vi "Measurement.UI.SetControllerDependency.vi"(8 "error in (no error)":errorcluster, 10 "Measurement":refnum<class "Measurement.lvclass">, 11 "Measurement.PhotocurrentMapping.UI in":refnum<class "Measurement.PhotocurrentMapping.UI.lvclass">) -> (0 "error out":errorcluster, 3 "Measurement.PhotocurrentMapping.UI out":refnum<class "Measurement.PhotocurrentMapping.UI.lvclass">)   [LabVIEW 2019, in "Measurement.PhotocurrentMapping.UI.lvclass"]
uses:
  Measurement.PhotocurrentMapping.UI.lvclass
  Measurement/Measurement.lvclass
  Measurement.PhotocurrentMapping/Measurement.PhotocurrentMapping.lvclass
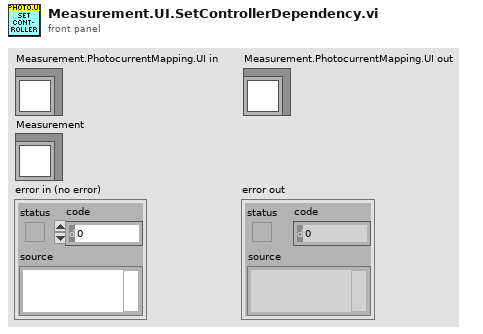
[diagram p1: front panel]
types:
  T1 = typedef "Measurement.PhotocurrentMapping.UI.lvclass/Dependencies--Cluster.ctl" = cluster{"Measurement.PhotocurrentMapping":refnum<class "Measurement.PhotocurrentMapping.lvclass">}
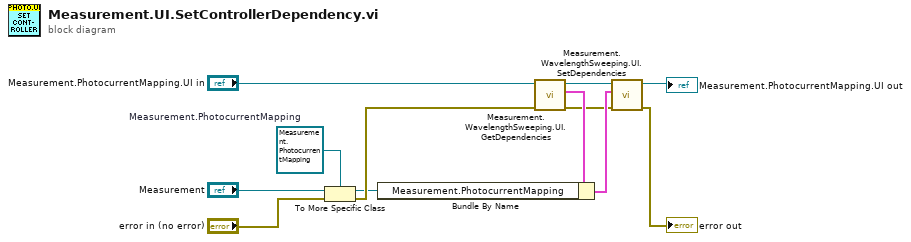
[diagram p0: block diagram]
diagram:
  w1 = refnum<class "Measurement.PhotocurrentMapping.lvclass"> refnum  # Measurement.PhotocurrentMapping
  n1 = To More Specific Class(target class=w1, reference="Measurement", error in="error in (no error)") -> (specific class reference=w7:refnum<class "Measurement.PhotocurrentMapping.lvclass">, error out=w9:errorcluster)
  n2 = call "Measurement.WavelengthSweeping.UI.GetDependencies.vi"("error in (no error)"=w9, "Measurement.PhotocurrentMapping.UI in"="Measurement.PhotocurrentMapping.UI in") -> ("error out"=w5:errorcluster, "Dependencies"=w8:T1, "Measurement.PhotocurrentMapping.UI out"=w4:refnum<class "Measurement.PhotocurrentMapping.UI.lvclass">)  [unwired: 7 in]
  n3 = Bundle By Name(cluster=w8, "Measurement.PhotocurrentMapping"=w7) -> (w6:T1)
  n4 = call "Measurement.WavelengthSweeping.UI.SetDependencies.vi"("error in (no error)"=w5, "Dependencies"=w6, "Measurement.PhotocurrentMapping.UI in"=w4) -> ("error out"=→"error out":errorcluster, "Measurement.PhotocurrentMapping.UI out"=→"Measurement.PhotocurrentMapping.UI out":refnum<class "Measurement.PhotocurrentMapping.UI.lvclass">)  [unwired: 7 in]
